vi "发送命令.vi"(1 "探头号":u8) -> (0 "探头命令":string)   [LabVIEW 2017]
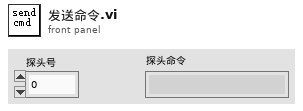
[diagram p1: front panel]
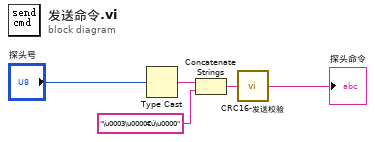
[diagram p0: block diagram]
diagram:
  n1 = Type Cast(x="探头号") -> (*(type *) &x=w3:string)  [unwired: 1 in]
  n2 = Concatenate Strings(w3, "\u0003\u0000€ú\u0000") -> (w2:string)
  n3 = call "CRC16-发送校验.vi"("净数据"=w2) -> ("完整输出"=→"探头命令":string)
